vi "Target.vi"() -> ()   [LabVIEW 2019]
uses:
  <vilib>/rvi/DataTransferAndStorage/Container/Common/niFpgaContainerExecOnDevCompGetState.vi
  <vilib>/rvi/Emulation/niFpgaEmulationIsFPGAContextNoSignature.vi
  <vilib>/rvi/Emulation/niFpgaSctlEmulationGetInTimedLoop.vi
  <vilib>/rvi/errors/niFpgaSetErrorForExecOnDevCompSimple.vi
  <vilib>/rvi/eio/common/nirviEmuReportErrorAndStop.vi
  <vilib>/rvi/DataTransferAndStorage/Container/Common/niFpgaContainerGetUniqueNameForEmu.vi
  <vilib>/rvi/FIFO/Fifo_Resource/nirvififoEmulationSetSize.vi
  <vilib>/rvi/FIFO/Fifo_Resource/nirviFifoEmulationQueueMgr.vi
  <instcachedir>/0/nirviFifoEmulationQueueMgr_E5CAEC123FF24DC58D834DCA3CDAA9B5.lvgen/nirviFifoEmulationQueueMgr_E5CAEC123FF24DC58D834DCA3CDAA9B5_005.vi
  <vilib>/rvi/FIFO/Fifo_Resource/nirvififoEmulationDetermineInputValidOut.vi
  <vilib>/rvi/FIFO/Fifo_Resource/nirvififoEmulationCreateLock.vi
  <vilib>/rvi/Emulation/niFpgaProcessEmulError.vi
  <vilib>/rvi/FIFO/Fifo_Resource/nirvififoEmulationObtainLock.vi
  <vilib>/rvi/FIFO/Fifo_Resource/nirvififoEmulationReleaseLock.vi
  <vilib>/rvi/occurrence/nirviWaitOnOccurrenceBase.vi
  <vilib>/rvi/errors/nirviReportUnexpectedCaseInternalError.vi
  <vilib>/rvi/errors/nirviReportUnexpectedCaseInternalError (U32).vi
  <vilib>/Utility/error.llb/Clear Errors.vi
  <vilib>/rvi/interface/RandomDataEmulation/niFpgaRandomDataHandleErrors.vi
  <vilib>/rvi/DataTransferAndStorage/Container/XNode/niFpgaContainer.xnode
  <vilib>/rvi/FIFO/Fifo_Resource/niFpgaFifoEmulationRefIn.vi
panel:
  out "T4 us":u16 caption="Tick Count(Ticks)"
  out "T2 us":u16 caption="Tick Count(mSec)"
  out "T3 us":u16 caption="Tick Count(mSec)"
  out "T5 us":u16 caption="crap"
  out "T1 us":u16 caption="Tick Count(mSec)"
  out "T5 ticks":u32 caption="Tick Count(mSec)"
  out "T4 tick":u32 caption="Tick Count(mSec)"
  out "T3 tick":u32 caption="Tick Count(mSec)"
  out "T2 tick":u32 caption="Tick Count(mSec)"
  out "T1 tick":u32 caption="Tick Count(mSec)"
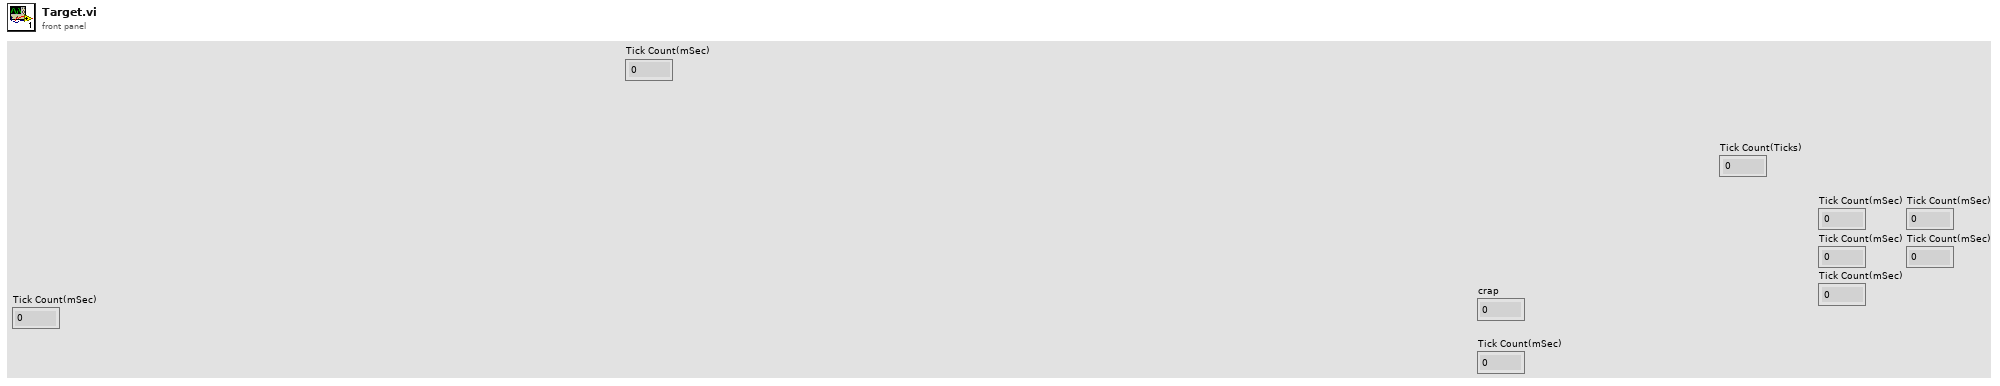
[diagram p1: front panel]
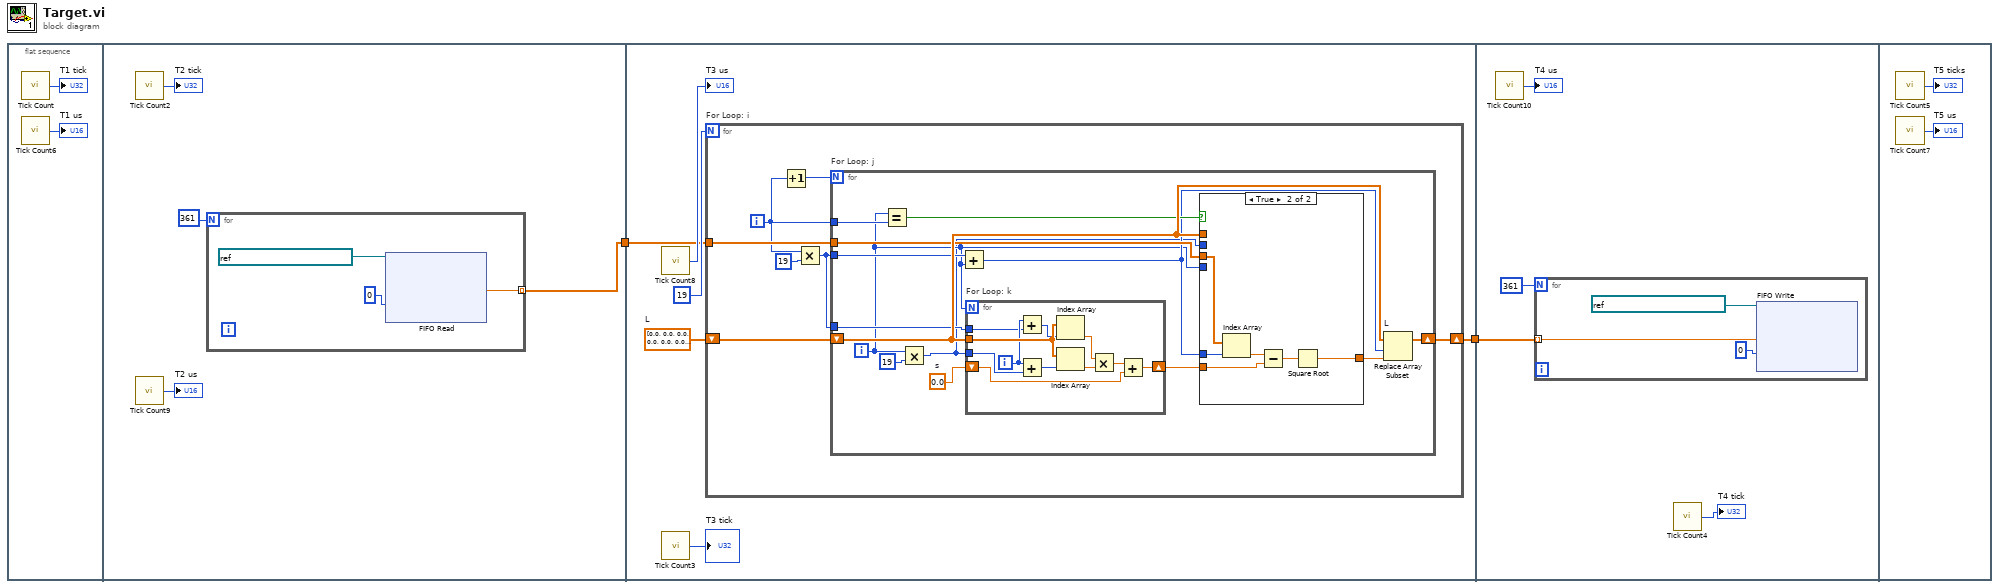
[diagram p0: block diagram]
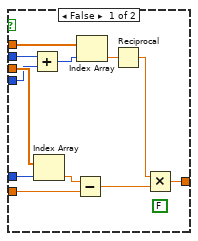
[diagram p2: hidden frame]
diagram:
  n1 = flat-sequence {
    tunnel: [w5] -> w2
    tunnel: w2 -> [w13]
    tunnel: [w12] -> w1
    tunnel: w1 -> [w69]
    frame #0 {
      n2 = call "Tick Count"() -> ("Tick Count(Ticks)"=→"T1 tick":u32)
      n3 = call "Tick Count6"() -> ("Tick Count(uSec)"=→"T1 us":u16)
    }
    frame #1 {
      n4 = call "Tick Count2"() -> ("Tick Count(Ticks)"=→"T2 tick":u32)
      n5 = call "Tick Count9"() -> ("Tick Count(uSec)"=→"T2 us":u16)
      n6 = for {
        N: 361 -> [_]
        tunnel: [w9] -> w5 mode=indexing
        n7 = xnode ("FIFO Read")("Timeout"=0, "FIFO In"=refnum<k21> "FIFO-host-to-Cholesky") -> ("Element"=w9:sgl)  [unwired: 2 out]
      }
    }
    frame #2 {
      w15 = sgl[] [0.0, 0.0, 0.0, 0.0, 0.0, 0.0, 0.0, 0.0, 0.0, 0.0, 0.0, 0.0, 0.0, 0.0, 0.0, 0.0, 0.0, 0.0, 0.0, 0.0, 0.0, 0.0, 0.0, 0.0, 0.0, 0.0, 0.0, 0.0, 0.0, 0.0, 0.0, 0.0, 0.0, 0.0, 0.0, 0.0, 0.0, 0.0, 0.0, 0.0, 0.0, 0.0, 0.0, 0.0, 0.0, 0.0, 0.0, 0.0, 0.0, 0.0, 0.0, 0.0, 0.0, 0.0, 0.0, 0.0, 0.0, 0.0, 0.0, 0.0, 0.0, 0.0, 0.0, 0.0, 0.0, 0.0, 0.0, 0.0, 0.0, 0.0, 0.0, 0.0, 0.0, 0.0, 0.0, 0.0, 0.0, 0.0, 0.0, 0.0, 0.0, 0.0, 0.0, 0.0, 0.0, 0.0, 0.0, 0.0, 0.0, 0.0, 0.0, 0.0, 0.0, 0.0, 0.0, 0.0, 0.0, 0.0, 0.0, 0.0, 0.0, 0.0, 0.0, 0.0, 0.0, 0.0, 0.0, 0.0, 0.0, 0.0, 0.0, 0.0, 0.0, 0.0, 0.0, 0.0, 0.0, 0.0, 0.0, 0.0, 0.0, 0.0, 0.0, 0.0, 0.0, 0.0, 0.0, 0.0, 0.0, 0.0, 0.0, 0.0, 0.0, 0.0, 0.0, 0.0, 0.0, 0.0, 0.0, 0.0, 0.0, 0.0, 0.0, 0.0, 0.0, 0.0, 0.0, 0.0, 0.0, 0.0, 0.0, 0.0, 0.0, 0.0, 0.0, 0.0, 0.0, 0.0, 0.0, 0.0, 0.0, 0.0, 0.0, 0.0, 0.0, 0.0, 0.0, 0.0, 0.0, 0.0, 0.0, 0.0, 0.0, 0.0, 0.0, 0.0, 0.0, 0.0, 0.0, 0.0, 0.0, 0.0, 0.0, 0.0, 0.0, 0.0, 0.0, 0.0, 0.0, 0.0, 0.0, 0.0, 0.0, 0.0, 0.0, 0.0, 0.0, 0.0, 0.0, 0.0, 0.0, 0.0, 0.0, 0.0, 0.0, 0.0, 0.0, 0.0, 0.0, 0.0, 0.0, 0.0, 0.0, 0.0, 0.0, 0.0, 0.0, 0.0, 0.0, 0.0, 0.0, 0.0, 0.0, 0.0, 0.0, 0.0, 0.0, 0.0, 0.0, 0.0, 0.0, 0.0, 0.0, 0.0, 0.0, 0.0, 0.0, 0.0, 0.0, 0.0, 0.0, 0.0, 0.0, 0.0, 0.0, 0.0, 0.0, 0.0, 0.0, 0.0, 0.0, 0.0, 0.0, 0.0, 0.0, 0.0, 0.0, 0.0, 0.0, 0.0, 0.0, 0.0, 0.0, 0.0, 0.0, 0.0, 0.0, 0.0, 0.0, 0.0, 0.0, 0.0, 0.0, 0.0, 0.0, 0.0, 0.0, 0.0, 0.0, 0.0, 0.0, 0.0, 0.0, 0.0, 0.0, 0.0, 0.0, 0.0, 0.0, 0.0, 0.0, 0.0, 0.0, 0.0, 0.0, 0.0, 0.0, 0.0, 0.0, 0.0, 0.0, 0.0, 0.0, 0.0, 0.0, 0.0, 0.0, 0.0, 0.0, 0.0, 0.0, 0.0, 0.0, 0.0, 0.0, 0.0, 0.0, 0.0, 0.0, 0.0, 0.0, 0.0, 0.0, 0.0, 0.0, 0.0, 0.0, 0.0, 0.0, 0.0, 0.0, 0.0, 0.0, 0.0, 0.0, 0.0, 0.0, 0.0, 0.0, 0.0, 0.0, 0.0, 0.0, 0.0, 0.0, 0.0, 0.0, 0.0, 0.0, 0.0, 0.0, 0.0, 0.0, 0.0, 0.0, 0.0, 0.0, 0.0, 0.0, 0.0, 0.0]  # L
      n8 = call "Tick Count8"() -> ("Tick Count(uSec)"=→"T3 us":u16)
      n9 = call "Tick Count3"() -> ("Tick Count(Ticks)"=→"T3 tick":u32)
      n10 = for "For Loop: i" {
        N: 19 -> [_]
        shift-right: [w22] -> w12
        shift-left: w15 -> [w24]
        tunnel: w13 -> [w21]
        i -> [w20]
        n11 = Increment(x=w20) -> (x+1=w23:i32)
        n12 = Multiply(x=w20, y=19) -> (x*y=w19:i32)
        n13 = for "For Loop: j" {
          N: w23 -> [_]
          tunnel: w20 -> [w34]
          shift-right: [w36] -> w22
          shift-left: w24 -> [w35]
          tunnel: w21 -> [w33]
          tunnel: w19 -> [w30]
          tunnel: w19 -> [w29]
          i -> [w28]
          w38 = sgl 0.0  # s
          n14 = Equal?(x=w28, y=w34) -> (x = y?=w32:bool)
          n15 = Multiply(x=w28, y=19) -> (x*y=w27:i32)
          n16 = Add(x=w30, y=w28) -> (x+y=w31:i32)
          n17 = for "For Loop: k" {
            N: w28 -> [_]
            tunnel: w35 -> [w67]
            shift-right: [w65] -> w37
            shift-left: w38 -> [w66]
            tunnel: w29 -> [w63]
            tunnel: w27 -> [w62]
            i -> [w64]
            n18 = Add(x=w64, y=w63) -> (x+y=w58:i32)
            n19 = Add(x=w64, y=w62) -> (x+y=w57:i32)
            n20 = Index Array(array=w67, index=w58) -> (element=w61:sgl)
            n21 = Index Array(array=w67, index=w57) -> (element=w60:sgl)
            n22 = Multiply(x=w61, y=w60) -> (x*y=w59:sgl)
            n23 = Add(x=w59, y=w66) -> (x+y=w65:sgl)
          }
          n24 = case shown="True" w32 {
            tunnel: w37 -> [w42 w56]
            tunnel: w35 -> [w50 _]
            tunnel: w33 -> [w47 w55]
            tunnel: w31 -> [w46 w54]
            tunnel: w28 -> [w45 _]
            tunnel: w27 -> [w44 _]
            tunnel: [w43 w52] -> w26
            frame False {
              (unwired) FALSE
              n25 = Add(x=w44, y=w45) -> (x+y=w40:i32)
              n26 = Index Array(array=w47, index=w46) -> (element=w39:sgl)
              n27 = Subtract(x=w39, y=w42) -> (x-y=w41:sgl)
              n28 = Index Array(array=w50, index=w40) -> (element=w49:sgl)
              n29 = Reciprocal(x=w49) -> (1/x=w48:sgl)
              n30 = Multiply(x=w48, y=w41) -> (x*y=w43:sgl)
            }
            frame True {
              n31 = Index Array(array=w55, index=w54) -> (element=w53:sgl)
              n32 = Subtract(x=w53, y=w56) -> (x-y=w51:sgl)
              n33 = Square Root(x=w51) -> (sqrt(x)=w52:sgl)
            }
          }
          n34 = Replace Array Subset "L"(array=w35, new element=w26, index=w31) -> (w36:sgl[])
        }
      }
    }
    frame #3 {
      n35 = call "Tick Count10"() -> ("Tick Count(uSec)"=→"T4 us":u16)
      n36 = for {
        N: 361 -> [_]
        tunnel: w69 -> [w74] mode=indexing
        n37 = xnode ("FIFO Write")("Element"=w74, "Timeout"=0, "FIFO In"=refnum<k21> "FIFO-Cholesky-to-host") -> ()  [unwired: 2 out]
      }
      n38 = call "Tick Count4"() -> ("Tick Count(Ticks)"=→"T4 tick":u32)
    }
    frame #4 {
      n39 = call "Tick Count5"() -> ("Tick Count(Ticks)"=→"T5 ticks":u32)
      n40 = call "Tick Count7"() -> ("Tick Count(uSec)"=→"T5 us":u16)
    }
  }
